vi "Configure ProgrammerTimer Action.vi"(0 "VISA resource name":refnum<visa-resource-name>, 1 "Unit Address (1)":u8=1 min=1 max=254, 9 "Timer/Programmer Action (0:SP)":u8(ring) items=["Servo from SP", "Servo from PV", "Ramp back from SP", "Ramp back from PV"], 11 "error in (no error)":errorcluster) -> (4 "VISA resource name out":refnum<visa-resource-name>, 15 "error out":errorcluster)   [LabVIEW 2010, in "Eurotherm 32xx Series.lvlib"]
doc: "This VI configures Program Setup Configuration Mode Parameters.\n\nWarning: This VI uses Controller Configuration Mode, this interrupts working process (device will not control).\nIt is recommended that the device should be disconnected from any active process."
uses:
  <instrlib>/Eurotherm 32xx Series/Eurotherm 32xx Series.lvlib
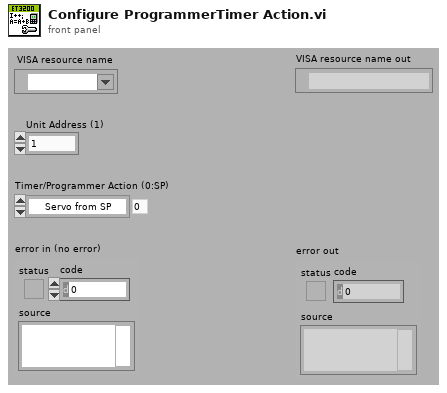
[diagram p1: front panel]
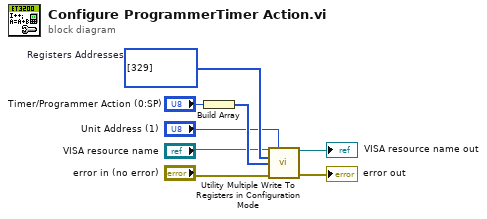
[diagram p0: block diagram]
diagram:
  w4 = u16[] [329]  # Registers Addresses
  n1 = Build Array("Timer/Programmer Action (0:SP)") -> (w5:u8[])
  n2 = call <instrlib>:"Utility Multiple Write To Registers in Configuration Mode.vi"("VISA resource name"="VISA resource name", "Unit Address (1)"="Unit Address (1)", "Registers Addresses (0)"=w4, "Data (0)"=w5, "error in (no error)"="error in (no error)") -> ("VISA resource name out"=→"VISA resource name out":refnum<visa-resource-name>, "error out"=→"error out":errorcluster)  [unwired: 9 in]
